vi "IntakeManager.vi"(10 "Intake":T1) -> ()   [LabVIEW 2014]
uses:
  IntakeControl.ctl
  Robot Global Data.vi
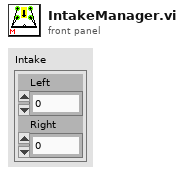
[diagram p1: front panel]
types:
  T1 = typedef "IntakeControl.ctl" = cluster{"Left":dbl, "Right":dbl}
  T2 = typedef "WPI_DigitalInputDevRef.ctl" = cluster{"DevStatus":errorcluster, "DIO Channel":T3, "Controller":T4}
  T3 = typedef "FPGA_DIOChannel.ctl" = enum8{"DIO 0", "DIO 1", "DIO 2", "DIO 3", "DIO 4", "DIO 5", "DIO 6", "DIO 7", "DIO 8", "DIO 9", "DIO MXP 0", "DIO MXP 1", "DIO MXP 2", "DIO MXP 3", "DIO MXP 4", "DIO MXP 5", "DIO MXP 6", "DIO MXP 7", "DIO MXP 8", "DIO MXP 9", "DIO MXP 10", "DIO MXP 11", "DIO MXP 12", "DIO MXP 13", "DIO MXP 14", "DIO MXP 15", "Invalid"}
  T4 = typedef "FPGA_TypedefDigitalModule.ctl" = enum16{"Controller 1"}
  T5 = typedef "WPI_MotorControlDeviceRef.ctl" = cluster{"DeviceStatus":errorcluster, "Type":T6, "PWM":cluster{"Controller":T4, "PWM Channel":T7, "DeadBand":T8}, "CAN":cluster{"Device Number":u8, "Control Mode":T9, "Semaphore":T10, "Max Vout":dbl, "TalonSRX Control Mode":T11}, "Invert":bool, "TransformRef":T12, "InvTransformRef":T12}
  T6 = typedef "WPI_MotorControlType.ctl" = enum16{"PWM", "CAN", "CANTalonSRX"}
  T7 = typedef "FPGA_DIOPWMChannel.ctl" = enum8{"PWM 0", "PWM 1", "PWM 2", "PWM 3", "PWM 4", "PWM 5", "PWM 6", "PWM 7", "PWM 8", "PWM 9", "PWM MXP 0", "PWM MXP 1", "PWM MXP 2", "PWM MXP 3", "PWM MXP 4", "PWM MXP 5", "PWM MXP 6", "PWM MXP 7", "PWM MXP 8", "PWM MXP 9", "Invalid"}
  T8 = typedef "WPI_PWMDeadband.ctl" = cluster{"Name":string, "maxPositivePwm":i32, "minPositivePwm":i32, "centerPwm":i32, "maxNegativePwm":i32, "minNegativePwm":i32, "angularRange":u16}
  T9 = typedef "WPI_CANJaguar_ControlMode.ctl" = enum8{"Percent VBus", "Current", "Speed", "Position", "Voltage"}
  T10 = typedef "Semaphore RefNum" = refnum<k1>
  T11 = typedef "WPI_CANTalonSRX_APIControlMode.ctl" = enum8{"Percent VBus", "Speed", "Position", "Slave", "Unchanged / Invalid"}
  T12 = typedef "WPI_PWMTransform_ConPane.ctl" = refnum<vi>
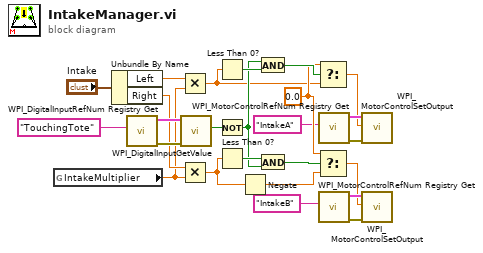
[diagram p0: block diagram]
diagram:
  w17 = 0.0
  n1 = global read "Robot Global Data.vi" "IntakeMultiplier"() -> (w3:dbl)
  n2 = Unbundle By Name("Intake") -> ("Left"=w5:dbl, "Right"=w4:dbl)
  n3 = call <vilib>:"WPI_DigitalInputRefNum Registry Get.vi"("refnum name"="TouchingTote") -> ("error out"=w24:errorcluster, "DigitalInputDevRef"=w23:T2)  [unwired: 9 in]
  n4 = Multiply(x=w5, y=w3) -> (x*y=w7:dbl)
  n5 = Multiply(x=w4, y=w3) -> (x*y=w1:dbl)
  n6 = call <vilib>:"WPI_DigitalInputGetValue.vi"("error in (no error)"=w24, "DigitalInputDevRef"=w23) -> ("Value"=w22:bool)  [unwired: 7 in, 2 out]
  n7 = Less Than 0?(x=w7) -> (x < 0?=w21:bool)
  n8 = Not(x=w22) -> (.not. x?=w18:bool)
  n9 = Less Than 0?(x=w1) -> (x < 0?=w19:bool)
  n10 = Negate(x=w1) -> (-x=w2:dbl)
  n11 = And(x=w18, y=w21) -> (x .and. y?=w20:bool)
  n12 = And(x=w19, y=w18) -> (x .and. y?=w16:bool)
  n13 = Select(t=w17, s=w20, f=w7) -> (s? t:f=w8:dbl)
  n14 = Select(t=w17, s=w16, f=w2) -> (s? t:f=w9:dbl)
  n15 = call <vilib>:"WPI_MotorControlRefNum Registry Get.vi"("refnum name"="IntakeA") -> ("error out"=w11:errorcluster, "MotorControlDevRef"=w10:T5)  [unwired: 9 in]
  n16 = call <vilib>:"WPI_MotorControlRefNum Registry Get.vi"("refnum name"="IntakeB") -> ("error out"=w13:errorcluster, "MotorControlDevRef"=w12:T5)  [unwired: 9 in]
  n17 = call <vilib>:"WPI_MotorControlSetOutput.vi"("error in (no error)"=w11, "Output"=w8, "MotorControlDevRef"=w10) -> ()  [unwired: 6 in, 3 out]
  n18 = call <vilib>:"WPI_MotorControlSetOutput.vi"("error in (no error)"=w13, "Output"=w9, "MotorControlDevRef"=w12) -> ()  [unwired: 6 in, 3 out]
